vi "DBL Constant.vi"(8 "error in (no error)":errorcluster caption="错误输入（无错误）", 10 "格式字符串":string="%f", 11 "Name":string) -> (0 "error out":errorcluster, 3 "Value":dbl)   [LabVIEW 2013, in "Resource Constant.lvlib"]
uses:
  Resource Constant.lvlib
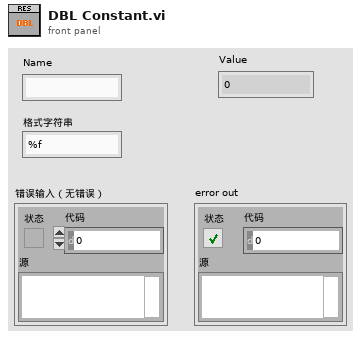
[diagram p1: front panel]
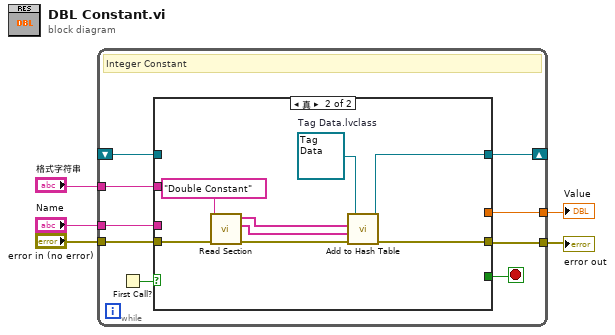
[diagram p0: block diagram]
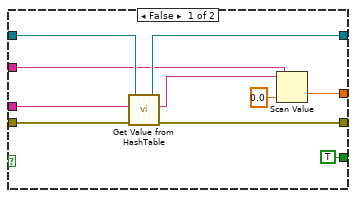
[diagram p2: hidden frame]
diagram:
  n1 = while {
    shift-right: [w11] -> _
    shift-left: _ -> [w10]
    tunnel: "error in (no error)" -> [w13]
    tunnel: [w12] -> w4
    tunnel: "Name" -> [w8]
    tunnel: [w7] -> w2
    tunnel: "格式字符串" -> [w6]
    stop <- w9 stop-if-true
    # "Integer Constant"
    n2 = First Call?() -> (First Call?: T/F=w14:bool)
    n3 = case shown="真" w14 {
      tunnel: w13 -> [w20 w29]
      tunnel: [w19 w27] -> w12
      tunnel: [w21 w26] -> w11
      tunnel: w10 -> [w23 _]
      tunnel: [TRUE _] -> w9
      tunnel: w8 -> [w22 _]
      tunnel: [w16 _] -> w7
      tunnel: w6 -> [w15 _]
      frame False {
        n4 = call-poly "Get Value from HashTable.vi"("error in (no error)"=w20, "Name"=w22, "Contstant Base 输入"=w23) -> ("error out"=w19:errorcluster, "Value"=w18:string, "Contstant Base 输出"=w21:refnum<class "Tag Data.lvclass">)  [unwired: 6 in]
        n5 = Scan Value(string=w18, format string=w15, default (0 dbl)=0.0 ("默认(0 dbl)")) -> (value=w16:dbl)  [unwired: 1 out]
      }
      frame True {
        w31 = refnum<class "Tag Data.lvclass"> refnum  # Tag Data.lvclass
        n6 = call "Read Section.vi"("error in (no error)"=w29, "section"="Double Constant") -> ("error out"=w28:errorcluster, "Value"=w25:string[], "key names"=w30:string[])  [unwired: 7 in]
        n7 = call-poly "Add to Hash Table.vi"("error in (no error)"=w28, "Value"=w25, "Name"=w30, "Contstant Base 输入"=w31) -> ("error out"=w27:errorcluster, "Contstant Base 输出"=w26:refnum<class "Tag Data.lvclass">)  [unwired: 6 in]
      }
    }
  }
  "error out" <- w4
  "Value" <- w2
